vi "Transmit TCPIP Packet.vi"(8 "error in (no error)":errorcluster, 10 "Packet":string, 11 "TCPIP Communications in":refnum<class "TCPIP Communications.lvclass">) -> (0 "error out":errorcluster, 3 "TCPIP Communications out":refnum<class "TCPIP Communications.lvclass">)   [LabVIEW 2015, in "TCPIP Communications Framework.lvlib" / "TCPIP Communications.lvclass"]
uses:
  TCPIP Communications.lvclass
  TCPIP Communications.lvclass/TCPIP Communications.ctl
  Utilities/Message Strings.llb/Message String Utilities.lvlib
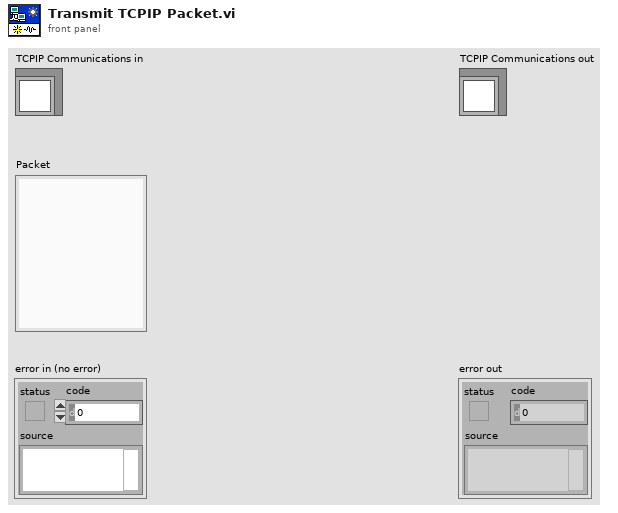
[diagram p1: front panel]
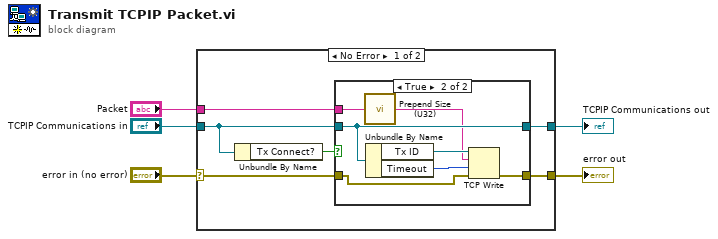
[diagram p0: block diagram]
diagram:
  n1 = case shown="No Error" "error in (no error)" {
    selector: "error in (no error)" -> [w9 w22]
    tunnel: [w6 w22] -> w1
    tunnel: [w8 w21] -> w2
    tunnel: "TCPIP Communications in" -> [w10 w21]
    tunnel: "Packet" -> [w7 _]
    frame No Error {
      n2 = Unbundle By Name(w10) -> ("Tx Connect?"=w11:bool)
      n3 = case shown="True" w11 {
        tunnel: w10 -> [w13 w20]
        tunnel: [w13 w20] -> w8
        tunnel: w9 -> [w12 w17]
        tunnel: [w12 w18] -> w6
        tunnel: w7 -> [_ w15]
        frame False {
        }
        frame True {
          n4 = call "Prepend Size (U32).vi"("String in"=w15) -> ("String out"=w14:string)
          n5 = Unbundle By Name(w20) -> ("Tx ID"=w19:refnum<k5>, "Timeout"=w16:i32)
          n6 = TCP Write(connection ID=w19, data in=w14, error in (no error)=w17, 9:w16) -> (error out=w18:errorcluster)  [unwired: 2 out]
        }
      }
    }
    frame Error {
    }
  }
  "error out" <- w1
  "TCPIP Communications out" <- w2
